vi "Bicoherence Analysis.vi"() -> ()   [LabVIEW 2023]
doc: "This example shows how to compute the bicoherence of a univariate time series using the TSA Bicoherence VI.\n\n<b>Instructions:</b>\n1) Run this VI.\n2) Make sure <B>Phase coupled? (T)</B> is set to TRUE.\n3) Observe that there are obvious peaks on the bicoherence graph.\n4) Set <B>Phase coupled? (T)</B> to FALSE.\n5) Observe that the bicoherence graph does not have any obvious peaks after stabilization."
uses:
  <vilib>/Native 3D Graph/xcontrol/3DPC_SurfacePlot.xctl
  <vilib>/measure/maspectr.llb/FFT Power Spectrum and PSD for 1 Chan.vi
  <vilib>/addons/Time Series Analysis/Correlation and Spectral Analysis.llb/TSA Bicoherence (Waveform).vi
  <vilib>/addons/_Advanced Signal Processing/NI_AdvSigProcTSA.lvlib
  <vilib>/measure/NI_MABase.lvlib
  <vilib>/measure/NI_MAPro.lvlib
panel:
  out "Power Spectrum":cluster{"f0":dbl, "df":dbl, "magnitude":dbl[]}(graph)
  in  "Phase coupled? (T)":bool=TRUE
  in  "Amplitude 3":dbl=1.0 format="%_4g"
  in  "Frequency 3":dbl=10.0 format="%_4g"
  in  "Amplitude 2":dbl=1.0 format="%_4g"
  in  "Frequency 2":dbl=6.0 format="%_4g"
  in  "Amplitude 1":dbl=1.0 format="%_4g"
  in  "Frequency 1":dbl=4.0 format="%_4g"
  in  "Noise variance":dbl=1.0 format="%_4g"
  in  "Window info":T1={"Window"=0, "Length"=128, "Overlap (%)"=0.0} {"Window" items=["None ", "Hanning", "Hamming", "Blackman-Harris", "Exact Blackman", "Blackman", "Flat Top", "4 Term B-Harris ", "7 Term B-Harris", "Low Sidelobe"]}
  out "aspt-left-top":bool
  in  "stop":bool
  in  "Frequency bins":i32=256
  out "Signal":waveform(dbl)(graph)
  out "Bicoherence":refnum<class "Base Datatype.lvclass">[](xcontrol)
  # "Overview: Shows how to compute the bicoherence of a univariate time series using the TSA Bicoherence VI.\nRequirements: LabVIEW Full Development System, Advanced Signal Processing Toolkit\nInstructions: \n1. Run this VI.\n2. Make sure Phase coupled? (T) is set to TRUE.\n3. Observe that there are obvious peaks on the bicoherence graph.\n4. Set Phase coupled? (T) to FALSE.\n5. Observe that the bicoherence graph does not have any obvious peaks after stabilization. \n6. Click Stop to stop the VI."
  # "Signal Settings"
  # "Bicoherence Settings"
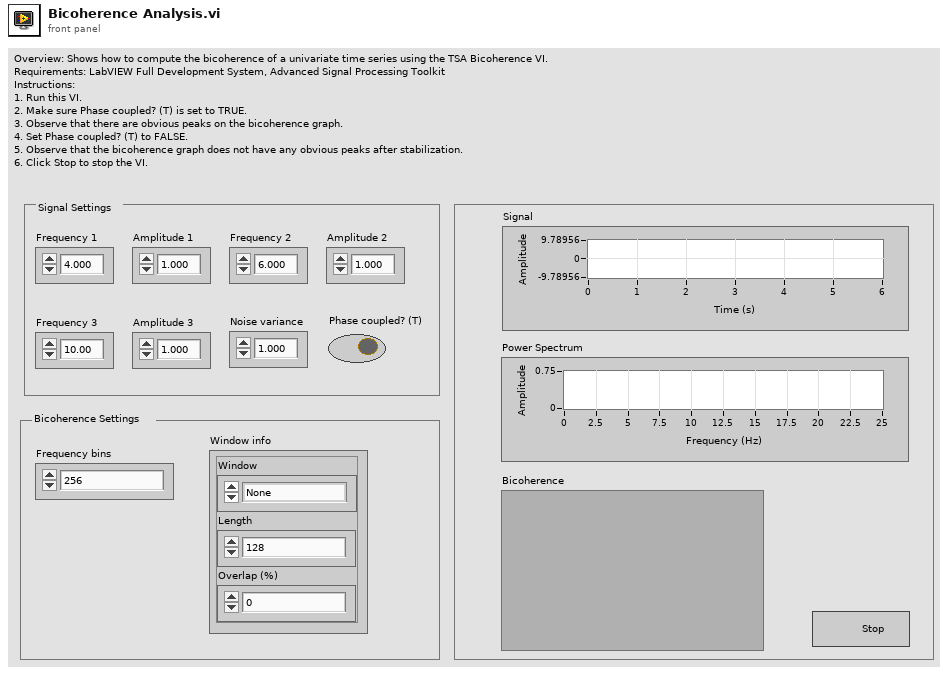
[diagram p1: front panel]
types:
  T1 = cluster{"Window":u16, "Length":i32, "Overlap (%)":dbl}
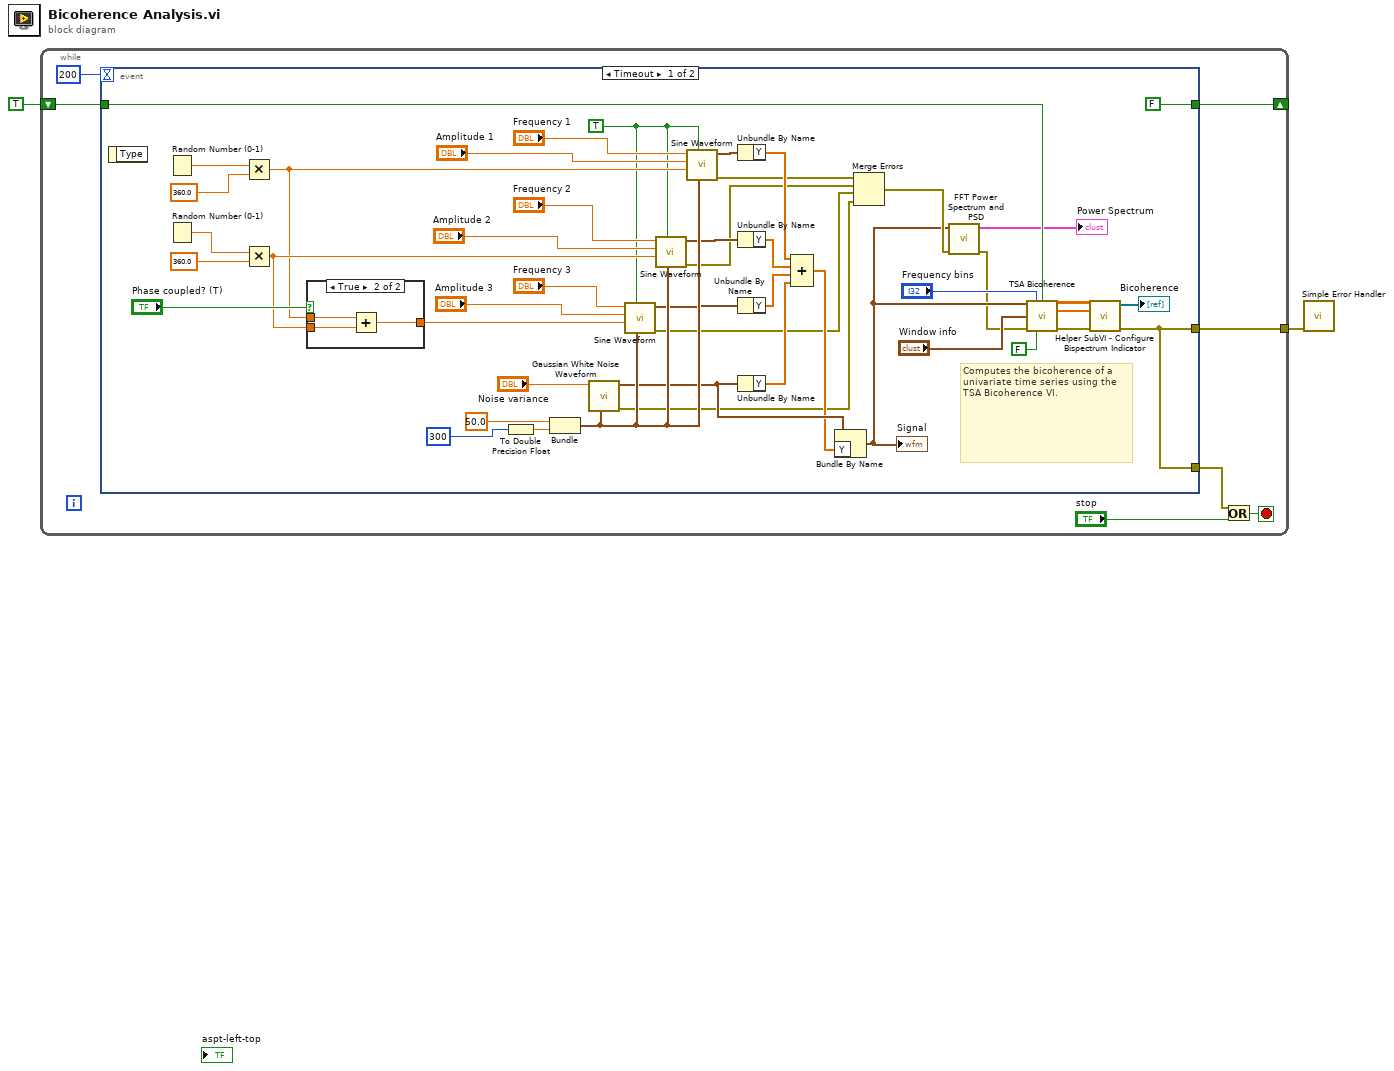
[diagram p0: block diagram]
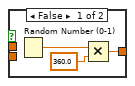
[diagram p2: hidden frame]
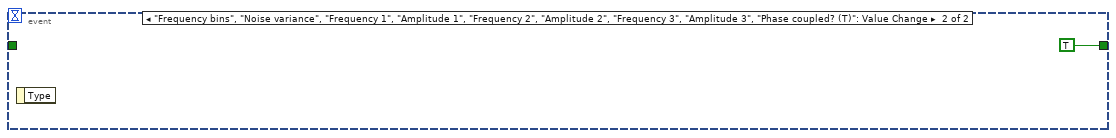
[diagram p3: hidden frame]
diagram:
  n1 = while {
    shift-right: [w5] -> _
    shift-left: TRUE ("initialize? (F)") -> [w6]
    tunnel: [w4] -> w1
    stop <- w8 stop-if-true
    n2 = event shown="[0] Timeout" {
      selector: _ -> [_ _]
      dyn-events: _ -> [_ _]
      timeout: 200 -> [_ _]
      tunnel: w6 -> [w24 _]
      tunnel: [FALSE ("initialize? (F)") TRUE ("initialize? (F)")] -> w5
      tunnel: [w15 _] -> w4
      tunnel: [w15 _] -> w3
      event Timeout {
        w37 = TRUE ("reset signal")
        # "Computes the bicoherence of a univariate time series using the TSA Bicoherence VI."
        n3 = event-data() -> ()  [unwired: 1 in, 1 out]
        n4 = Random Number (0-1)() -> (number: 0 to 1=w56:dbl)
        n5 = Random Number (0-1)() -> (number: 0 to 1=w51:dbl)
        n6 = Multiply(x=w56, y=360.0) -> (x*y=w46:dbl)
        n7 = Multiply(x=w51, y=360.0) -> (x*y=w47:dbl)
        n8 = case shown="True" "Phase coupled? (T)" {
          tunnel: w47 -> [_ w62]
          tunnel: w46 -> [_ w61]
          tunnel: [w57 w60] -> w45
          frame False {
            n9 = Random Number (0-1)() -> (number: 0 to 1=w58:dbl)
            n10 = Multiply(x=w58, y=360.0) -> (x*y=w57:dbl)
          }
          frame True {
            n11 = Add(x=w61, y=w62) -> (x+y=w60:dbl)
          }
        }
        n12 = To Double Precision Float(number=300 ("#s")) -> (double precision float=w41:dbl)
        n13 = Bundle("Fs"=50.0, w41) -> (w38:cluster{"Fs":dbl, dbl})  [unwired: 1 out]
        n14 = call <vilib>:"Gaussian White Noise Waveform.vi"("sampling info"=w38, "standard deviation"="Noise variance") -> ("error out"=w16:errorcluster, "signal out"=w29:waveform(dbl))  [unwired: 3 in, 5 out]
        n15 = call <vilib>:"Sine Waveform.vi"("sampling info"=w38, "reset signal"=w37, "phase"=w45, "amplitude"="Amplitude 3", "frequency"="Frequency 3") -> ("error out"=w17:errorcluster, "signal out"=w34:waveform(dbl))  [unwired: 2 in, 3 out]
        n16 = call <vilib>:"Sine Waveform.vi"("sampling info"=w38, "reset signal"=w37, "phase"=w47, "amplitude"="Amplitude 2", "frequency"="Frequency 2") -> ("error out"=w18:errorcluster, "signal out"=w35:waveform(dbl))  [unwired: 2 in, 3 out]
        n17 = call <vilib>:"Sine Waveform.vi"("sampling info"=w38, "reset signal"=w37, "phase"=w46, "amplitude"="Amplitude 1", "frequency"="Frequency 1") -> ("error out"=w19:errorcluster, "signal out"=w36:waveform(dbl))  [unwired: 2 in, 3 out]
        n18 = Unbundle By Name(w36) -> ("Y"=w33:dbl[])
        n19 = Unbundle By Name(w35) -> ("Y"=w32:dbl[])
        n20 = Unbundle By Name(w34) -> ("Y"=w31:dbl[])
        n21 = Unbundle By Name(w29) -> ("Y"=w30:dbl[])
        n22 = Compound Arithmetic op=ADD(w33, w32, w31, w30) -> (w28:dbl[])
        n23 = Bundle By Name(cluster=w29, "Y"=w28) -> (w13:waveform(dbl))
        "Signal" <- w13
        n24 = Merge Errors(w19, w18, w17, w16) -> (w14:errorcluster)
        n25 = call-poly <vilib>:"FFT Power Spectrum and PSD.vi"("error in (no error)"=w14, "time signal"=w13) -> ("error out"=w11:errorcluster, "Power Spectrum / PSD"=→"Power Spectrum":cluster{"f0":dbl, "df":dbl, "magnitude":dbl[]})  [unwired: 6 in, 2 out]
        n26 = call-poly <vilib>:"TSA Bicoherence.vi"("Xt"=w13, "frequency bins"="Frequency bins", "initialize? (F)"=w24, "window info"="Window info", "error in (no error)"=w11, "dB on? (T)"=FALSE ("dB on? (F)")) -> ("S(f,f)"=w22:dbl[][], "freq bins"=w21:dbl[], "error out"=w20:errorcluster)  [unwired: 7 in]
        n27 = call "Helper SubVI - Configure Bispectrum Indicator.vi"("error in (no error)"=w20, "frequency bins"=w21, "S(f,f)"=w22) -> ("error out"=w15:errorcluster, "bispectrum  indicator"=→"Bicoherence":refnum<class "Base Datatype.lvclass">[])  [unwired: 7 in]
      }
      event "Frequency bins", "Noise variance", "Frequency 1", "Amplitude 1", "Frequency 2", "Amplitude 2", "Frequency 3", "Amplitude 3", "Phase coupled? (T)", "Window info.Window", "Window info.Length", "Window info.Overlap (%)": Value Change {
        n28 = event-data() -> ()  [unwired: 1 in, 1 out]
      }
    }
    n29 = Or(x=w3, y="stop") -> (x .or. y?=w8:bool)
  }
  n30 = call <vilib>:"Simple Error Handler.vi"("error in (no error)"=w1) -> ()  [unwired: 1 in, 8 out]
